vi "dialog_wait.vi"(7 "dialog type (single line)":T1, 8 "error in":errorcluster, 10 "title string":string="Please wait ...", 11 "message string":string="Please wait, generating report ...") -> (0 "error out":errorcluster, 3 "reference out":refnum<vi>)   [LabVIEW 2013, in "varilib.lvlib"]
doc: "Assynchronously calls wait dialog with custom message."
uses:
  varilib.lvlib
  dialog_wait_type.ctl
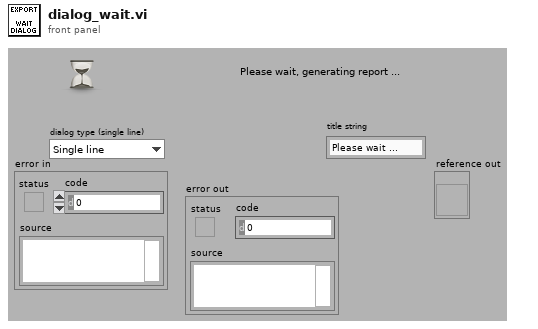
[diagram p1: front panel]
types:
  T1 = typedef "varilib.lvlib/dialog_wait_type.ctl" = enum16{"Single line", "Multi line"}
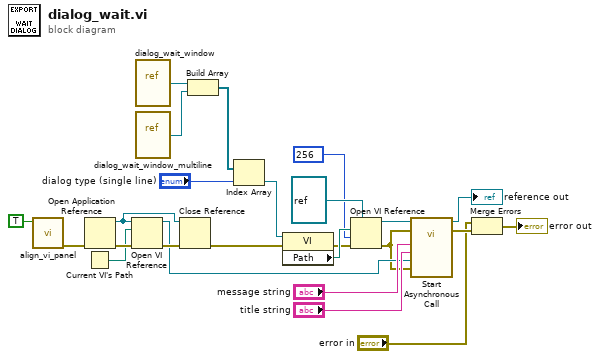
[diagram p0: block diagram]
diagram:
  n1 = call "align_vi_panel.vi"("use top level VI (T)"=TRUE) -> ("error out"=w14:errorcluster)  [unwired: 10 in]
  n2 = Open Application Reference(8:w14) -> (0:w18:errorcluster, 3:w16:refnum<vi>)  [unwired: 3 in]
  n3 = Current VI's Path() -> (path=w15:path)
  n4 = Open VI Reference(application reference (local)=w16, vi path=w15, error in (no error)=w18) -> (vi reference=w10:refnum<vi>, error out=w17:errorcluster)  [unwired: 3 in]
  n5 = vi-ref "dialog_wait_window.vi"() -> (w5:refnum<vi>)
  n6 = vi-ref "dialog_wait_window_multiline.vi"() -> (w4:refnum<vi>)
  n7 = Close Reference(reference=w16, error in (no error)=w17) -> (error out=w13:errorcluster)
  n8 = Build Array(w5, w4) -> (w3:refnum<vi>[])
  n9 = Index Array(array=w3, index="dialog type (single line)") -> (element=w1:refnum<vi>)
  n10 = property class="VI"(reference=w1, error in=w13) -> (error out=w22:errorcluster, "Path"=w25:path)  [unwired: 1 out]
  n11 = Open VI Reference(type specifier VI Refnum (for type only)=refnum<vi> refnum, vi path=w25, options=256, error in (no error)=w22) -> (vi reference=w23:refnum<vi>, error out=w9:errorcluster)  [unwired: 2 in]
  n12 = call-by-ref "Start Asynchronous Call"(reference=w23, error in=w9, "error in"=w9, "top vi reference"=w10, "title"="title string", "msg"="message string") -> (reference out=→"reference out":refnum<vi>, error out=w21:errorcluster)  [unwired: 7 in, 1 out]
  n13 = Merge Errors("error in", w21) -> (→"error out":errorcluster)
